vi "Counting Inputs.vi"(8 "error in (no error)":errorcluster, 9 "j (0)":T1, 10 "i (0)":T2, 11 "VISA resource name":refnum<visa-resource-name>) -> (0 "error out":errorcluster, 3 "VISA resource name out":refnum<visa-resource-name>)   [LabVIEW 2015, in "SR400.lvlib"]
doc: "CI i { ,j }\nThe CI command sets and reads the counter\ninputs. i = 0, 1, or 2 selecting counter A,B, or T\nand is required. If j is included, then the input to\ncounter i is changed to source j. If j is absent, the\ninput to counter i is returned.\nj Input\n0 10 MHz\n1 INPUT 1\n2 INPUT 2\n3 TRIG\nCounter Allowed Inputs\nA 10 MHz, INPUT1\nB INPUT 1, INPUT 2\nT 10 MHz, INPUT 2, TRIG\nChanging a counter input while counting may\nresult in bad count data."
uses:
  SR400.lvlib
  Typedefs/Counter.ctl
  Typedefs/Counting Input.ctl
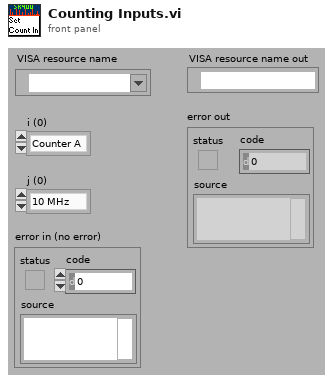
[diagram p1: front panel]
types:
  T1 = typedef "SR400.lvlib/Counting Input.ctl" = enum16{"10 MHz", "INPUT 1", "INPUT 2", "TRIG"}
  T2 = typedef "SR400.lvlib/Counter.ctl" = enum16{"Counter A", "Counter B", "Counter T"}
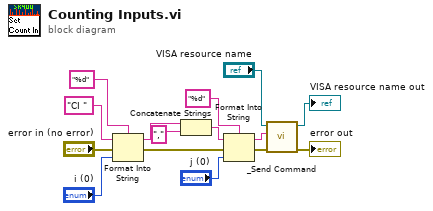
[diagram p0: block diagram]
diagram:
  n1 = Format Into String(format string="%d", initial string="CI " ("command"), error in="error in (no error)", "i (0)") -> (resulting string=w12:string, error out=w13:errorcluster)
  n2 = Concatenate Strings(w12, "," ("command")) -> (w7:string)
  n3 = Format Into String(format string="%d", initial string=w7, error in=w13, "j (0)") -> (resulting string=w4:string, error out=w3:errorcluster)
  n4 = call "_Send Command.vi"("error in (no error)"=w3, "Command"=w4, "VISA resource name"="VISA resource name") -> ("error out"=→"error out":errorcluster, "VISA resource name out"=→"VISA resource name out":refnum<visa-resource-name>)  [unwired: 1 in, 6 out]
